vi "Home Actuator.vi"(8 "error in (no error)":errorcluster, 11 "VISA resource name":refnum<visa-resource-name>) -> (0 "error out":errorcluster, 3 "VISA resource name out":refnum<visa-resource-name>)   [LabVIEW 2018]
doc: "Moves the actuator to position 1. If the actuator is already in position 1, the command is ignored.\n\n\n(Nimble Focus Consulting 2019)"
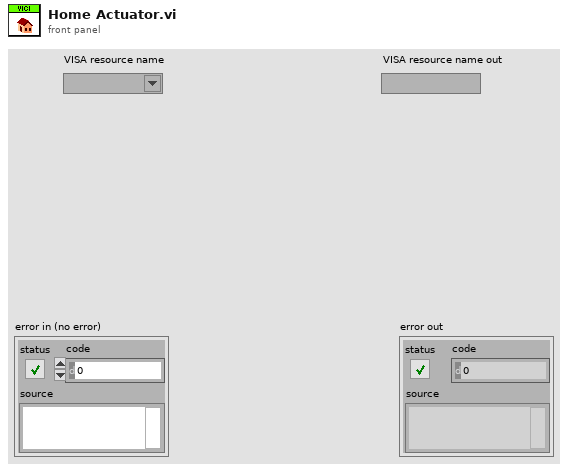
[diagram p1: front panel]
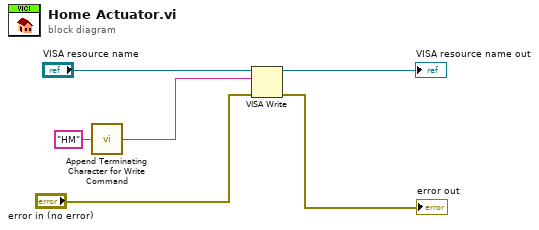
[diagram p0: block diagram]
diagram:
  n1 = call "Append Terminating Character for Write Command.vi"("Command in"="HM") -> ("Command with Terminating character out"=w2:string)
  n2 = VISA Write(VISA resource name="VISA resource name", write buffer=w2, error in (no error)="error in (no error)") -> (VISA resource name out=→"VISA resource name out":refnum<visa-resource-name>, error out=→"error out":errorcluster)  [unwired: 1 out]
